vi "get_data.vi"(0 "Analog_Input.lvclass (in)":refnum<class "Analog_Input.lvclass">, 11 "error in":errorcluster) -> (4 "Analog_Input.lvclass":refnum<class "Analog_Input.lvclass">, 15 "error out":errorcluster)   [LabVIEW 2013, in "Analog_Input.lvclass"]
uses:
  Analog_Input.lvclass
  Analog_Input.lvclass/Analog_Input.ctl
  <vilib>/DAQmx/read.llb/DAQmx Read (Analog 2D DBL NChan NSamp).vi
  Globals.vi
  <vilib>/DAQmx/miscellaneous.llb/DAQmx Fill In Error Info.vi
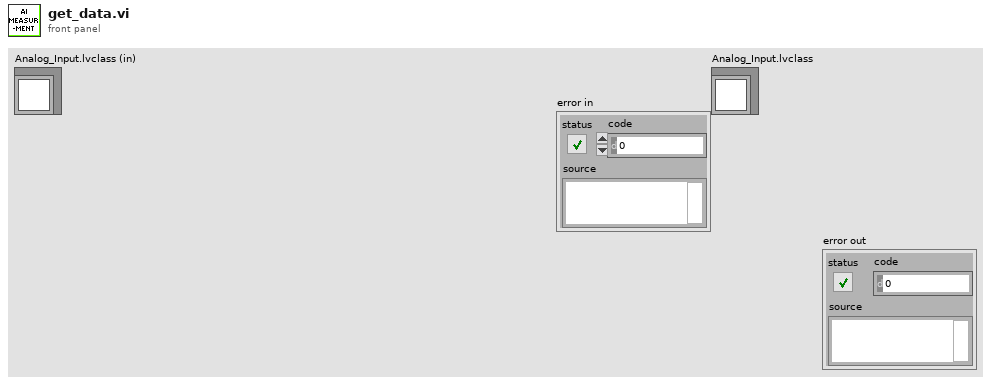
[diagram p1: front panel]
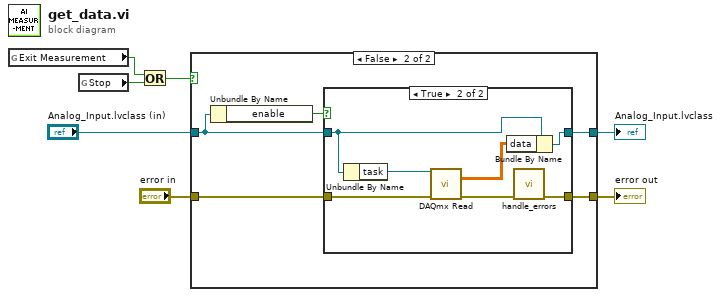
[diagram p0: block diagram]
diagram:
  n1 = global read "Globals.vi" "Exit Measurement"() -> (w6:bool)
  n2 = global read "Globals.vi" "Stop"() -> (w5:bool)
  n3 = Or(x=w6, y=w5) -> (x .or. y?=w4:bool)
  n4 = case shown="False" w4 {
    tunnel: "error in" -> [w9 w12]
    tunnel: [w9 w10] -> w1
    tunnel: "Analog_Input.lvclass (in)" -> [w8 w13]
    tunnel: [w8 w11] -> w2
    frame True {
    }
    frame False {
      n5 = Unbundle By Name(w13) -> ("enable"=w14:bool)
      n6 = case shown="True" w14 {
        tunnel: w13 -> [w16 w20]
        tunnel: w12 -> [w15 w22]
        tunnel: [w16 w21] -> w11
        tunnel: [w15 w17] -> w10
        frame False {
        }
        frame True {
          n7 = Unbundle By Name(w20) -> ("task"=w23:refnum<k21>)
          n8 = call-poly <vilib>:"DAQmx Read.vi"("task/channels in"=w23, "error in"=w22) -> ("data"=w19:dbl[][], "error out"=w18:errorcluster)  [unwired: 11 in, 1 out]
          n9 = Bundle By Name(cluster=w20, "data"=w19) -> (w21:refnum<class "Analog_Input.lvclass">)
          n10 = call "handle_errors.vi"("error in (no error)"=w18) -> ("error out"=w17:errorcluster)  [unwired: 14 in]
        }
      }
    }
  }
  "error out" <- w1
  "Analog_Input.lvclass" <- w2
